vi "NStageMRate Decimation Filter.vi"   [LabVIEW 2023]
doc: "----------------------\n\nThis filter is configured as follows:\n\n<b>Filter Configuration</b>\nOverall type: Multirate - Decimation\nOverall Factor: 100\nNumber of stages: 3\n\n <b>Stage 1</b>\n Type: Multirate - Decimation\n Structure: Polyphase FIR\n Factor: 10\n\n <b>Stage 2</b>\n Type: Multirate - Decimation\n Structure: Polyphase FIR\n Factor: 5\n\n <b>Stage 3</b>\n Type: Multirate - Decimation\n Structure: Polyphase FIR\n Factor: 2\n\n<b>Input Data Type</b>\nType: fixed-point <±,16,1> [-1.000000E+0,9.999695E-1]:3.051758E-5\n\n<b>Output Data Type</b>\nType: fixed-point <±,16,4> [-8.000000E+0,7.999756E+0]:2.441406E-4\nRounding mode: Round-Half-Even\nOverflow mode: Saturate\n\n<b>Implementation</b>\nNumber of channels: 1\nMaximum input sampling rate per channel @ 40MHz: 10MHz\nGain processing: On Host\n\n<b>Execution Mode</b>\nOutside single-cycle Timed Loop\nThroughput: 4 cycles/sample"
uses:
  <vilib>/Platform/TimedLoop/XDataNode/timing_clust.ctl
  <vilib>/Platform/TimedLoop/XDataNode/nitl_modes.ctl
  <vilib>/Platform/TimedLoop/XDataNode/wakeup.ctl
  <vilib>/rvi/Emulation/niFpgaSctlEmulationGetInTimedLoop.vi
  <vilib>/Utility/error.llb/Clear Errors.vi
  <vilib>/rvi/Emulation/niFpgaEmulationIsFPGAContextNoSignature.vi
  <vilib>/rvi/errors/niFpgaSetErrorForExecOnDevCompSimple.vi
  <vilib>/rvi/eio/common/nirviEmuReportErrorAndStop.vi
  <vilib>/rvi/DataTransferAndStorage/Container/Common/niFpgaContainerGetUniqueNameForEmu.vi
  <vilib>/rvi/FIFO/Fifo_Resource/nirvififoEmulationSetSize.vi
  <vilib>/rvi/FIFO/Fifo_Resource/nirviFifoEmulationQueueMgr.vi
  <instcachedir>/0/nirviFifoEmulationQueueMgr_E5CAEC123FF24DC58D834DCA3CDAA9B5.lvgen/nirviFifoEmulationQueueMgr_E5CAEC123FF24DC58D834DCA3CDAA9B5_002.vi
  <vilib>/rvi/FIFO/Fifo_Resource/nirvififoEmulationCreateLock.vi
  <vilib>/rvi/Emulation/niFpgaProcessEmulError.vi
  <vilib>/rvi/FIFO/Fifo_Resource/nirvififoEmulationObtainLock.vi
  <vilib>/rvi/FIFO/Fifo_Resource/nirvififoEmulationReleaseLock.vi
  <vilib>/rvi/occurrence/nirviWaitOnOccurrenceBase.vi
  <vilib>/rvi/errors/nirviReportUnexpectedCaseInternalError.vi
  <vilib>/rvi/errors/nirviReportUnexpectedCaseInternalError (U32).vi
  <instcachedir>/0/nirviFifoEmulationQueueMgr_E5CAEC123FF24DC58D834DCA3CDAA9B5.lvgen/nirviFifoEmulationQueueMgr_E5CAEC123FF24DC58D834DCA3CDAA9B5_007.vi
  <vilib>/rvi/FIFO/Fifo_Resource/nirvififoEmulationDetermineInputValidOut.vi
  <vilib>/Platform/TimedLoop/XDataNode/XDataNode.xnode
  <vilib>/rvi/DataTransferAndStorage/Container/XNode/niFpgaContainer.xnode
  <vilib>/rvi/FIFO/Fifo_Resource/nirvififoEmulationRead.vi
  <vilib>/rvi/FIFO/Fifo_Resource/nirvififoEmulationWrite.vi
  <vilib>/Platform/TimedLoop/XDataNode/XDNodeRunTimeDep.lvlib
types:
  T1 = typedef "XDNodeRunTimeDep.lvlib/timing_clust.ctl" = cluster{"Expected End [f-1]":u64, "Actual End [f-1]":u64, "Finished Late? [f-1]":bool, "Expected End [i-1]":u64, "Actual End [i-1]":u64, "Finished Late? [i-1]":bool, "Expected Start [i]":u64, "Actual Start [i]":u64, "Expected Start [f]":u64, "Actual Start [f]":u64, "Source Name":string, "Structure Name":string, "Period":i64, "Deadline":i64, "Offset":i64, "Start":i64, "Priority":i32, "Timeout":i32, "Mode":T2, "Wakeup Reason":T3, "Error":errorcluster, "Source Type":string, "Secondary Source Type":string, "Global End Time":u64, "Global Start Time":u64, "Frame Duration":u64, "Iteration Duration":u64, "Assigned CPU":i32, "I/O Scan Engine Mode":u32}
  T2 = typedef "XDNodeRunTimeDep.lvlib/nitl_modes.ctl" = enum32{"No Change", "Process missed periods, maintain original phase", "Discard missed periods, maintain original phase", "Process missed periods, ignore original phase", "Discard missed periods, ignore original phase"}
  T3 = typedef "XDNodeRunTimeDep.lvlib/wakeup.ctl" = enum32{"Normal", "Aborted", "Asynchronous wakeup", "Timing source error", "Timed loop error", "Timeout"}
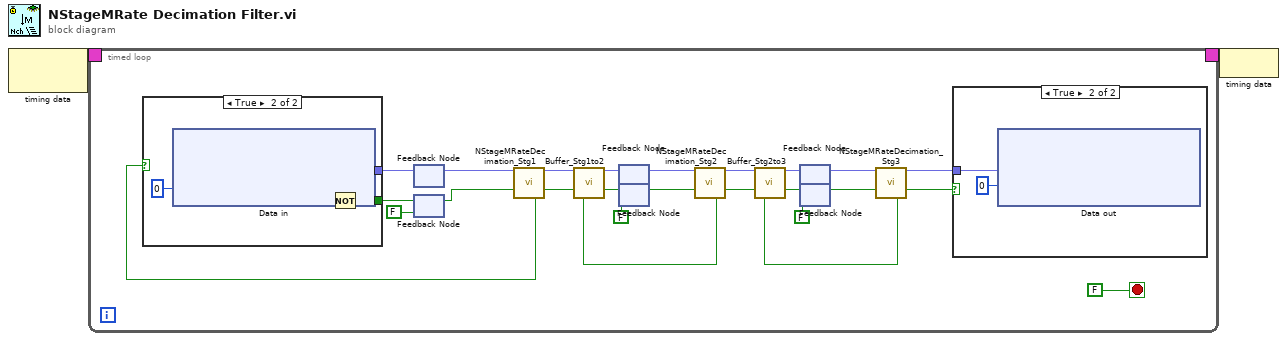
[diagram p0: block diagram]
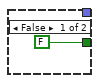
[diagram p3: hidden frame]
diagram:
  n1 = node-c288() -> (w2:T1)  [unwired: 1 in]
  n2 = timed-loop "Main Loop" {
    timing: w2 -> [_]
    timing-out: [_] -> w1
    stop <- FALSE stop-if-true
    n3 = feedback #1() -> (w21:fxp<+/-,16,1>)  [unwired: 1 out]
    n4 = feedback #2(FALSE) -> (w24:bool)
    n5 = call "NStageMRateDecimation_Stg1"("input data"=w21, "input valid"=w24) -> ("output data"=w18:fxp<+/-,32,2>, "output valid"=w17:bool, "ready for input"=w22:bool)  [unwired: 11 in]
    n6 = case "DataInCase" shown="True" w22 {
      tunnel: [_ w33] -> w27
      tunnel: [FALSE w31] -> w26
      frame False {
      }
      frame True {
        n7 = xnode ("Data in")("Timeout"=0) -> ("Element"=w33:fxp<+/-,16,1>, "Timed Out?"=w32:bool)  [unwired: 1 in, 1 out]
        n8 = Not(x=w32) -> (.not. x?=w31:bool)
      }
    }
    n9 = feedback-in #1(w27) -> ()
    n10 = feedback-in #2(w26) -> ()
    n11 = feedback #3() -> (w13:fxp<+/-,32,2>)  [unwired: 1 in]
    n12 = feedback #4(FALSE) -> (w12:bool)
    n13 = call "NStageMRateDecimation_Stg2"("input data"=w13, "input valid"=w12) -> ("output data"=w10:fxp<+/-,32,3>, "output valid"=w9:bool, "ready for input"=w11:bool)  [unwired: 11 in]
    n14 = call "Buffer_Stg1to2"("input data"=w18, "input valid"=w17, "ready for output"=w11) -> ("output data"=w14:fxp<+/-,32,2>, "output valid"=w16:bool)  [unwired: 11 in]
    n15 = feedback-in #3(w14) -> ()
    n16 = feedback-in #4(w16) -> ()
    n17 = feedback #5() -> (w5:fxp<+/-,32,3>)  [unwired: 1 in]
    n18 = feedback #6(FALSE) -> (w4:bool)
    n19 = call "NStageMRateDecimation_Stg3"("input data"=w5, "input valid"=w4) -> ("output data"=w20:fxp<+/-,16,4>, "output valid"=w19:bool, "ready for input"=w3:bool)  [unwired: 11 in]
    n20 = call "Buffer_Stg2to3"("input data"=w10, "input valid"=w9, "ready for output"=w3) -> ("output data"=w6:fxp<+/-,32,3>, "output valid"=w8:bool)  [unwired: 11 in]
    n21 = feedback-in #5(w6) -> ()
    n22 = feedback-in #6(w8) -> ()
    n23 = case "DataOutCase" shown="True" w19 {
      tunnel: w20 -> [_ w29]
      frame False {
      }
      frame True {
        n24 = xnode ("Data out")("Element"=w29, "Timeout"=0) -> ()  [unwired: 1 in, 2 out]
      }
    }
  }
  n25 = node-c288(w1) -> ()
